vi "Shutdown.vi"(8 "error in (no error)":errorcluster, 11 "Abstract Consumer in":refnum<class "Abstract Consumer.lvclass">) -> (0 "error out":errorcluster, 3 "Abstract Consumer out":refnum<class "Abstract Consumer.lvclass">)   [LabVIEW 2027, in "Messaging.lvlib" / "Abstract Consumer.lvclass"]
uses:
  Abstract Consumer.lvclass
  Abstract Consumer.lvclass/Abstract Consumer.ctl
  Message Queue/Abstract Message Queue/Abstract Message Queue.lvclass
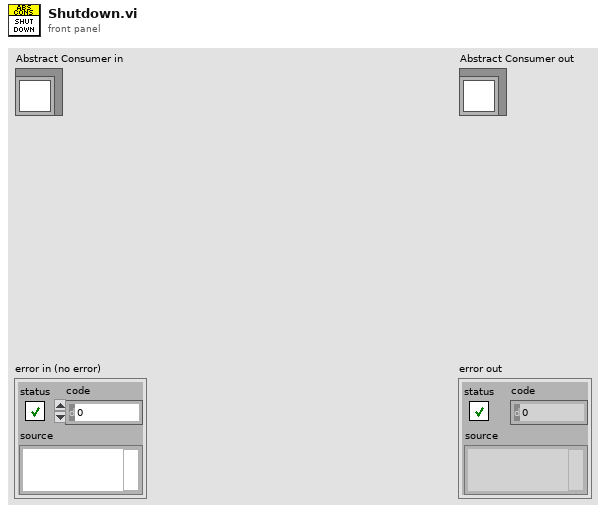
[diagram p1: front panel]
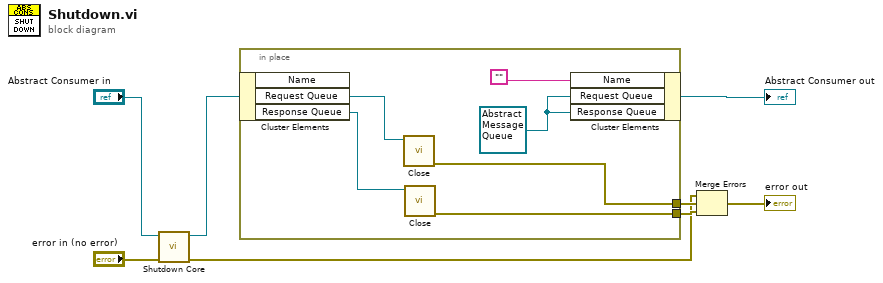
[diagram p0: block diagram]
diagram:
  n1 = call-dynamic "Shutdown Core.vi"("error in (no error)"="error in (no error)", "Abstract Consumer in"="Abstract Consumer in") -> ("error out"=w3:errorcluster, "Abstract Consumer out"=w1:refnum<class "Abstract Consumer.lvclass">)  [unwired: 8 in]
  n2 = in-place {
    in-place-border: [w10] -> w6
    in-place-border: [w9] -> w5
    w11 = refnum<class "Abstract Message Queue.lvclass"> refnum ("Request Queue")
    n3 = in-place-cluster #1(w1) -> ("Request Queue"=w13:refnum<class "Abstract Message Queue.lvclass">, "Response Queue"=w12:refnum<class "Abstract Message Queue.lvclass">)  [unwired: 1 out]
    n4 = call-dynamic "Close.vi"("Abstract Message Queue in"=w13) -> ("error out"=w10:errorcluster)  [unwired: 9 in, 1 out]
    n5 = call-dynamic "Close.vi"("Abstract Message Queue in"=w12) -> ("error out"=w9:errorcluster)  [unwired: 9 in, 1 out]
    n6 = in-place-cluster #1("Name"="", "Request Queue"=w11, "Response Queue"=w11) -> (→"Abstract Consumer out":refnum<class "Abstract Consumer.lvclass">)
  }
  n7 = Merge Errors(w3, w6, w5) -> (→"error out":errorcluster)
